vi "Init MCP.vi"(8 "error in (no error)":errorcluster, 11 "Data Cluster in":T1) -> (0 "error out":errorcluster, 3 "Data Cluster out":T1)   [LabVIEW 2026, in "G-AI Core.lvlib"]
uses:
  G-AI Core.lvlib
  Module Data--cluster.ctl
  <vilib>/jgoebel/LabVIEW MCP Server SDK/MCP Server.lvlib
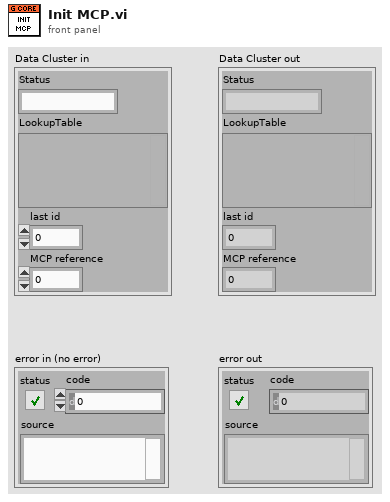
[diagram p1: front panel]
types:
  T1 = typedef "G-AI Core.lvlib/Module Data--cluster.ctl" = cluster{"Status":string, "LookupTable":variant, "last id":i32, "MCP reference":i32}
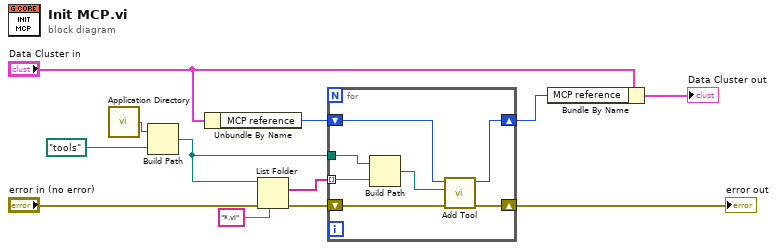
[diagram p0: block diagram]
diagram:
  n1 = call <vilib>:"Application Directory.vi"() -> ("Application Directory"=w7:path)
  n2 = Build Path(base path=w7, name or relative path=path "tools") -> (appended path=w4:path)
  n3 = Unbundle By Name("Data Cluster in") -> ("MCP reference"=w10:i32)
  n4 = List Folder(path=w4, pattern="*.vi", error in="error in (no error)") -> (filenames=w3:string[], error out=w5:errorcluster)  [unwired: 1 in, 2 out]
  n5 = for {
    shift-right: [w19] -> w11
    shift-left: w5 -> [w17]
    tunnel: w4 -> [w16]
    tunnel: w3 -> [w15] mode=indexing
    shift-right: [w13] -> w1
    shift-left: w10 -> [w18]
    n6 = Build Path(base path=w16, name or relative path=w15) -> (appended path=w14:path)
    n7 = call <vilib>:"Add Tool.vi"("error in (no error)"=w17, "vi path"=w14, "server id"=w18) -> ("error out"=w19:errorcluster, "server id out"=w13:i32)  [unwired: 7 in]
  }
  "error out" <- w11
  n8 = Bundle By Name(cluster="Data Cluster in", "MCP reference"=w1) -> (→"Data Cluster out":T1)
